vi "LSX Get Key.vi"(0 "lLSID":i32, 1 "pbKey4":i32, 5 "pbKey1":i32, 7 "pbKey2":i32, 9 "pbKey3":i32, 11 "error in (no error)":errorcluster) -> (3 "pbKey4 out":i32, 4 "function return":i32, 6 "pbKey1 out":i32, 8 "pbKey2 out":i32, 10 "pbKey3 out":i32, 15 "error out":errorcluster)   [LabVIEW 2016, in "Tango_DLL.lvlib"]
doc: "TANGOAPI int TANGOCALL LSX_GetKey (int lLSID, BOOL *pbKey1, BOOL *pbKey2, BOOL *pbKey3, BOOL *pbKey4);"
uses:
  Tango_DLL.lvlib
  2017/Microscope Control/Device Library/Stages/Marzhauser/SCAN IM 120 x 80/Tango DLL VIs/Tango_DLL.dll
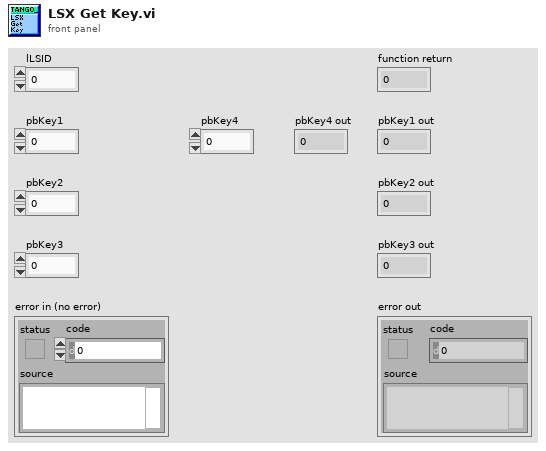
[diagram p1: front panel]
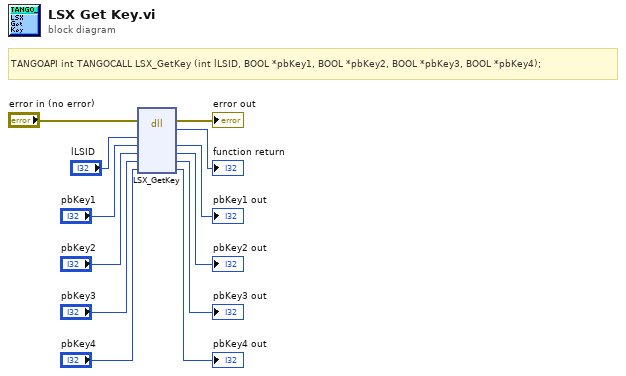
[diagram p0: block diagram]
diagram:
  # "TANGOAPI int TANGOCALL LSX_GetKey (int lLSID, BOOL *pbKey1, BOOL *pbKey2, BOOL *pbKey3, BOOL *pbKey4);"
  n1 = dll-call lib="C:/Users/4PiSMS/Documents/Microscope Control/2017/Microscope Control/Device Library/Stages/Marzhauser/SCAN IM 120 x 80/Tango DLL VIs/Tango_DLL.*" fn="LSX_GetKey"(error in="error in (no error)", "lLSID"="lLSID", "pbKey1"="pbKey1", "pbKey2"="pbKey2", "pbKey3"="pbKey3", "pbKey4"="pbKey4") -> (error out=→"error out":errorcluster, →"function return":i32, "pbKey1"=→"pbKey1 out":i32, "pbKey2"=→"pbKey2 out":i32, "pbKey3"=→"pbKey3 out":i32, "pbKey4"=→"pbKey4 out":i32)  [unwired: 3 in, 1 out]
